vi "Get SLSC Switch Capabilities Version.vi"(8 "error in (no error)":errorcluster, 11 "SLSC Switch Custom Device Ref in":T1 format="%.0x") -> (0 "error out":errorcluster, 2 "Capabilities Version":string, 3 "SLSC Switch Custom Device Ref out":T1 format="%.0x")   [LabVIEW 2020]
uses:
  SLSC Scripting Constants.vi
  SLSC Switch Scripting.lvlib
  <vilib>/NI VeriStand/Custom Device API/Custom Device API.lvlib
  <vilib>/NI VeriStand/Custom Device API/Get Item Property (String).vi
  <vilib>/NI VeriStand/Custom Device API/Custom Device Item Ref.ctl
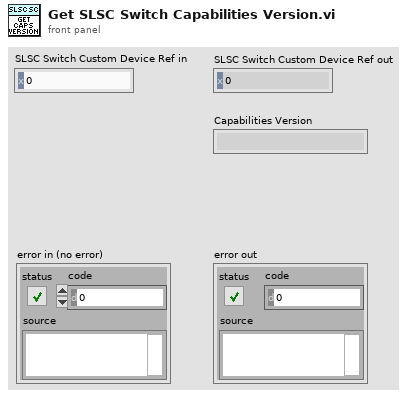
[diagram p1: front panel]
types:
  T1 = typedef "Custom Device API.lvlib/Custom Device Item Ref.ctl" = u64
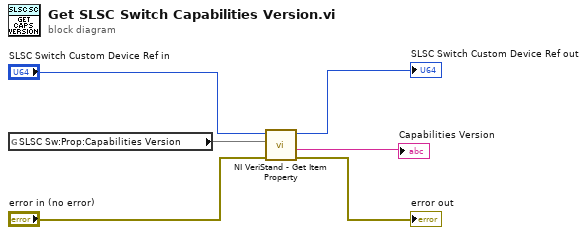
[diagram p0: block diagram]
diagram:
  n1 = global read "SLSC Scripting Constants.vi" "SLSC Sw:Prop:Capabilities Version"() -> (w3)
  n2 = call-poly <vilib>:"NI VeriStand - Get Item Property.vi"("error in (no error)"="error in (no error)", "Property Name"=w3, "Item Ref in"="SLSC Switch Custom Device Ref in") -> ("error out"=→"error out":errorcluster, "Value"=→"Capabilities Version":string, "Item Ref out"=→"SLSC Switch Custom Device Ref out":T1)  [unwired: 5 in, 1 out]
